vi "Pick Multiplier.vi"() -> ()   [LabVIEW 2009]
uses:
  Motor Control Global.vi
  Multiplier Enumeration.ctl
panel:
  out "Writing Index":u32
  out "FIFO":refnum<k21>
  out "Memory":refnum<k21>
  in  "Enum":T1
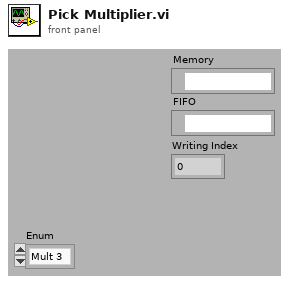
[diagram p1: front panel]
types:
  T1 = typedef "Multiplier Enumeration.ctl" = enum16{"Mult 3", "Mult 2", "Mult 1"}
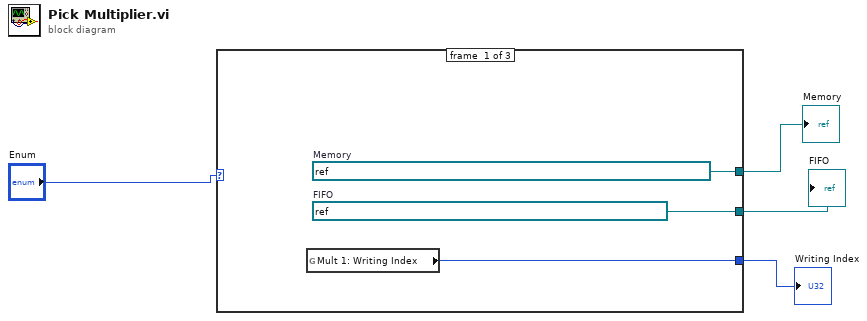
[diagram p0: block diagram]
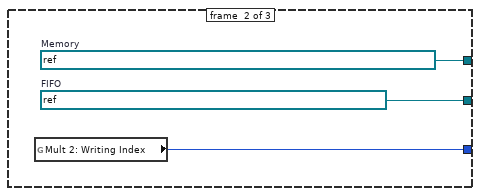
[diagram p2: hidden frame]
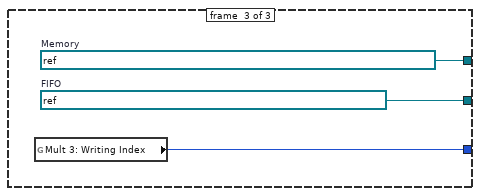
[diagram p3: hidden frame]
diagram:
  n1 = case shown="\"Mult 3\"" "Enum" {
    tunnel: [w7 w10 w13] -> w1
    tunnel: [w6 w9 w12] -> w2
    tunnel: [w5 w8 w11] -> w3
    frame #0 {
      w6 = refnum<k21> "Multiplier 1 FIFO In :  [8b Idendifier; 20b args; 18b fxp ; 18b fxp]"  # FIFO
      w5 = refnum<k21> "Multiplier 1 Block Memory Out : [8b Identifier; 6b args; 18b fxp output]"  # Memory
      n2 = global read "Motor Control Global.vi" "Mult 1: Writing Index"() -> (w7:u32)
    }
    frame #1 {
      w9 = refnum<k21> "Multiplier 2 FIFO In : [8b Identifier; 20b args; 18b fxp; 18b fxp]"  # FIFO
      w8 = refnum<k21> "Multiplier 2 Block Memory Out: [8b Identifier; 6b args; 18b fxp output]"  # Memory
      n3 = global read "Motor Control Global.vi" "Mult 2: Writing Index"() -> (w10:u32)
    }
    frame #2 {
      w12 = refnum<k21> "Multiplier 3 FIFO In : [8b Identifier; 20b args; 18b fxp; 18b fxp]"  # FIFO
      w11 = refnum<k21> "Multiplier 3 Block Memory Out: [8b Identifier; 6b args; 18b fxp output]"  # Memory
      n4 = global read "Motor Control Global.vi" "Mult 3: Writing Index"() -> (w13:u32)
    }
  }
  "Memory" <- w3
  "FIFO" <- w2
  "Writing Index" <- w1
